vi "Command Loop.vi"(8 "Error in":errorcluster, 10 "Queue Refs":T1, 11 "Device Reference in":T2 format="%.0x") -> ()   [LabVIEW 2025, in "Runtime Configuration Support Inline Async Example Engine.lvlib"]
uses:
  Runtime Configuration Support Inline Async Example Engine.lvlib
  <vilib>/NI VeriStand/Custom Device API/Custom Device Item Ref.ctl
  Shared/ReConfigured.Settings.ctl
  Shared/Compiled.Settings.ctl
  <vilib>/NI VeriStand/Custom Device API/Block Data Reference.ctl
  <vilib>/NI VeriStand/Custom Device API/Data Reference.ctl
  <vilib>/NI VeriStand/Custom Device API/Message Response (String).ctl
  <vilib>/NI VeriStand/Custom Device API/Message Response (Byte Array).ctl
  <vilib>/NI VeriStand/Custom Device API/Custom Device API.lvlib
  Shared/Runtime Configuration Support Inline Async Example Shared.lvlib
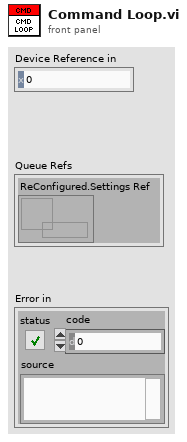
[diagram p1: front panel]
types:
  T1 = cluster{"ReConfigured.Settings Ref":refnum<queue>}
  T2 = typedef "Custom Device API.lvlib/Custom Device Item Ref.ctl" = u64
  T3 = typedef "Custom Device API.lvlib/Custom Device Engine Event Ref.ctl" = refnum<event-registration>
  T4 = typedef "Custom Device API.lvlib/Message Response (String).ctl" = cluster{"Response":string, "Error":errorcluster}
  T5 = typedef "Custom Device API.lvlib/Message Response (Byte Array).ctl" = cluster{"Response":u8[], "Error":errorcluster}
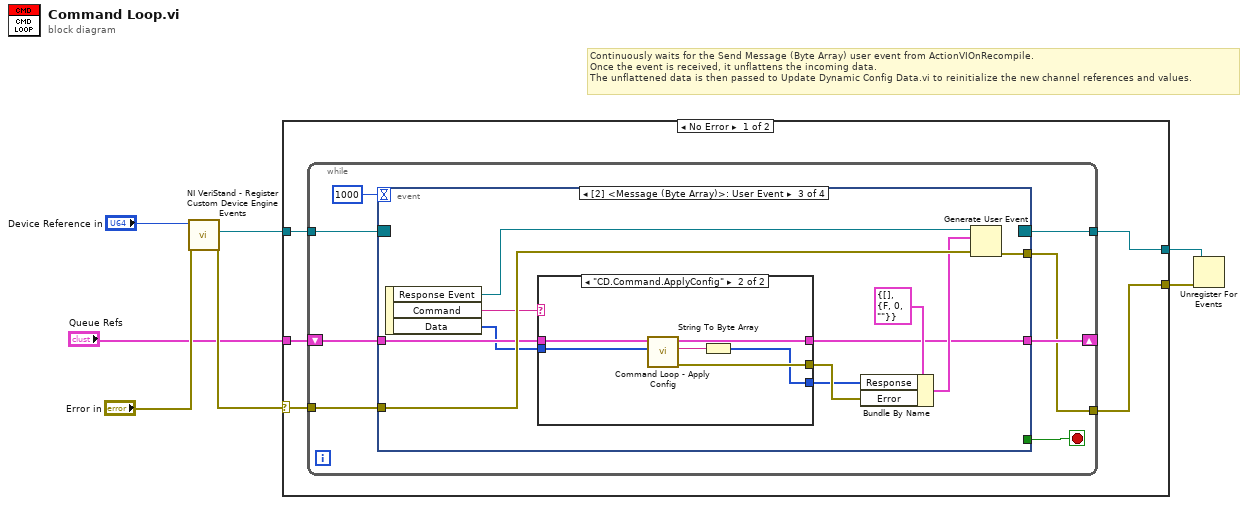
[diagram p0: block diagram]
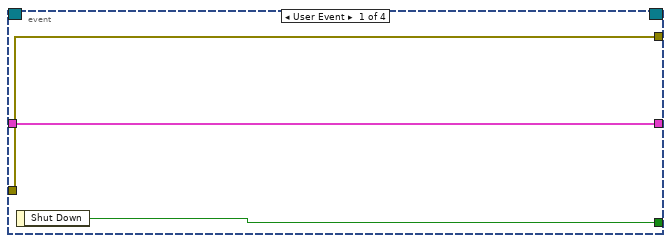
[diagram p2: hidden frame]
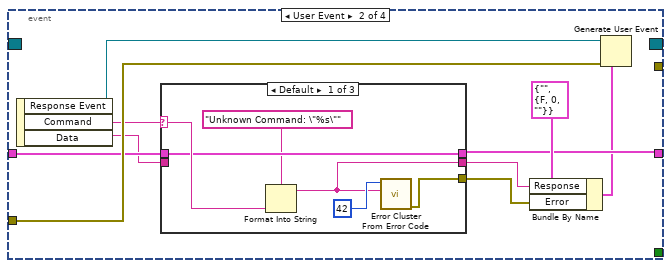
[diagram p3: hidden frame]
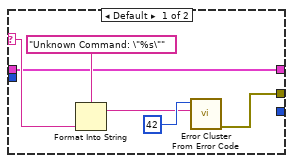
[diagram p6: hidden frame]
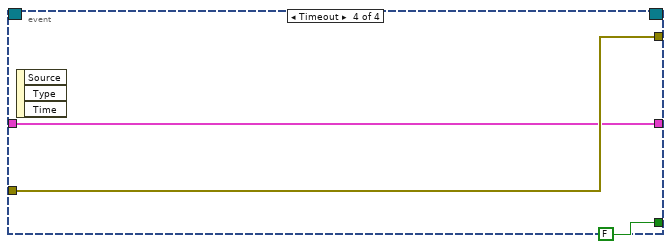
[diagram p7: hidden frame]
diagram:
  # "Continuously waits for the Send Message (Byte Array) user event from ActionVIOnRecompile.\nOnce the event is received, it unflattens the incoming data.\nThe unflattened data is then passed to Update Dynamic Config Data.vi to reinitialize the new channel references and values."
  n1 = call <vilib>:"NI VeriStand - Register Custom Device Engine Events.vi"("error in (no error)"="Error in", "Device Ref in"="Device Reference in") -> ("error out"=w5:errorcluster, "Custom Device Engine Event Ref"=w2:T3)  [unwired: 7 in, 1 out]
  n2 = case shown="No Error" w5 {
    selector: w5 -> [w9 w66]
    tunnel: [w12 _] -> w4
    tunnel: [w8 w66] -> w7
    tunnel: w2 -> [w11 _]
    tunnel: "Queue Refs" -> [w10 _]
    frame No Error {
      n3 = while {
        tunnel: [w19] -> w12
        tunnel: w11 -> [w18]
        shift-right: [w15] -> _
        shift-left: w10 -> [w16]
        tunnel: w9 -> [w14]
        tunnel: [w13] -> w8
        stop <- w20 stop-if-true
        n4 = event shown="[2] <Message (Byte Array)>: User Event" {
          selector: w18 -> [_ _ _ _]
          dyn-events: [_ _ _ _] -> w19
          timeout: 1000 -> [_ _ _ _]
          tunnel: [w22 _ _ FALSE ("Shut Down")] -> w20
          tunnel: [w23 _ w49 w65] -> w13
          tunnel: w14 -> [w23 w33 w48 w65]
          tunnel: w16 -> [w21 w28 w43 w63]
          tunnel: [w21 w27 w42 w63] -> w15
          event User Event {
            n5 = event-data() -> ("Shut Down"=w22:bool)  [unwired: 1 in]
          }
          event User Event {
            n6 = event-data() -> ("Response Event"=w29:refnum<user-event>, "Command"=w30:string, "Data"=w26:string)  [unwired: 1 in]
            n7 = case shown="Default" w30 {
              selector: w30 -> [w37 _ _]
              tunnel: w28 -> [w36 _ _]
              tunnel: [w36 _ _] -> w27
              tunnel: w26 -> [_ _ _]
              tunnel: [w34 _ _] -> w24
              tunnel: [w39 _ _] -> w32
              frame Default {
                n8 = Format Into String(format string="Unknown Command: \"%s\"", w37) -> (resulting string=w34:string)  [unwired: 2 in, 1 out]
                n9 = call <vilib>:"Error Cluster From Error Code.vi"("error message (\"\")"=w34, "error code (0)"=42) -> ("error out"=w39:errorcluster)  [unwired: 7 in]
              }
              frame "CD.Command.SetHWValues" {
              }
              frame "CD.Command.GetHWValues" {
              }
            }
            n10 = Bundle By Name(cluster=T4 {"Response"="", "Error"={"status"=FALSE, "code"=0, "source"=""}} ("event data"), "Response"=w24, "Error"=w32) -> (w25:T4)
            n11 = Generate User Event(user event=w29, event data cluster=w25, error in=w33) -> ()  [unwired: 1 in, 2 out]
          }
          event User Event {
            n12 = event-data() -> ("Response Event"=w47:refnum<user-event>, "Command"=w44:string, "Data"=w41:u8[])  [unwired: 1 in]
            n13 = case shown="\"CD.Command.ApplyConfig\"" w44 {
              selector: w44 -> [w53 _]
              tunnel: [w56 w62] -> w50
              tunnel: w43 -> [w51 w57]
              tunnel: [w51 w61] -> w42
              tunnel: w41 -> [_ w60]
              tunnel: [_ w59] -> w40
              frame Default {
                n14 = Format Into String(format string="Unknown Command: \"%s\"", w53) -> (resulting string=w52:string)  [unwired: 2 in, 1 out]
                n15 = call <vilib>:"Error Cluster From Error Code.vi"("error message (\"\")"=w52, "error code (0)"=42) -> ("error out"=w56:errorcluster)  [unwired: 7 in]
              }
              frame "CD.Command.ApplyConfig" {
                n16 = call "Command Loop - Apply Config.vi"("Data"=w60, "Queue Refs in"=w57) -> ("error out"=w62:errorcluster, "Response"=w58:string, "Queue Refs out"=w61:T1)  [unwired: 7 in]
                n17 = String To Byte Array(string=w58) -> (unsigned byte array=w59:u8[])
              }
            }
            n18 = Bundle By Name(cluster=T5 {"Response"=[], "Error"={"status"=FALSE, "code"=0, "source"=""}} ("event data"), "Response"=w40, "Error"=w50) -> (w45:T5)
            n19 = Generate User Event(user event=w47, event data cluster=w45, error in=w48) -> (error out=w49:errorcluster)  [unwired: 1 in, 1 out]
          }
          event Timeout {
            n20 = event-data() -> ()  [unwired: 1 in, 3 out]
          }
        }
      }
    }
    frame Error {
    }
  }
  n21 = Unregister For Events(event registration refnum=w4, error in=w7) -> ()  [unwired: 1 out]
